vi "VI Tree.vi"   [LabVIEW 2012, in "Phidget Stepper.lvlib"]
doc: "${Stepper:VITreeHeader}"
uses:
  <instrlib>/Phidgets/Phidget Stepper/Phidget Stepper.lvlib
  <instrlib>/Phidgets/Phidget Stepper/Public/StepperStart.vi
  <instrlib>/Phidgets/Phidget Stepper/Public/StepperOpen.vi
  <instrlib>/Phidgets/Phidget Stepper/Public/StepperClose.vi
panel:
  # "(c) 2015 Phidgets Inc..  ALL RIGHTS RESERVED."
  # "SEE DIAGRAM\nFOR VI TREE."
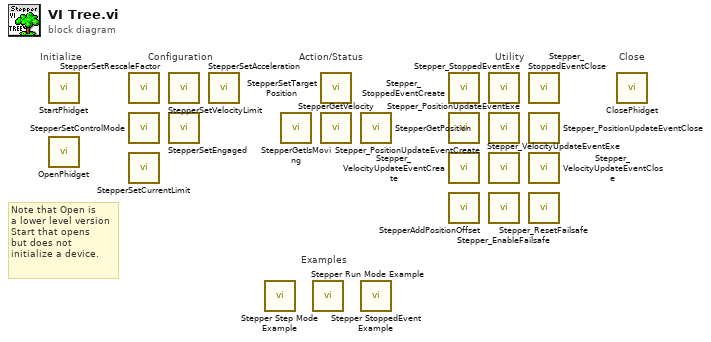
[diagram p0: block diagram]
diagram:
  # "Note that Open is\na lower level version\nStart that opens\nbut does not \ninitialize a device."
  # "Examples"
  # "Configuration"
  # "Utility"
  # "Action/Status"
  # "Close"
  # "Initialize"
  n1 = call-poly <instrlib>:"StartPhidget.vi"() -> ()  [unwired: 12 in, 4 out]
  n2 = call-poly <instrlib>:"OpenPhidget.vi"() -> ()  [unwired: 8 in, 4 out]
  n3 = call <instrlib>:"StepperSetRescaleFactor.vi"() -> ()  [unwired: 9 in, 2 out]
  n4 = call <instrlib>:"StepperSetControlMode.vi"() -> ()  [unwired: 9 in, 2 out]
  n5 = call <instrlib>:"StepperSetCurrentLimit.vi"() -> ()  [unwired: 9 in, 2 out]
  n6 = call <instrlib>:"StepperSetVelocityLimit.vi"() -> ()  [unwired: 9 in, 2 out]
  n7 = call <instrlib>:"StepperSetEngaged.vi"() -> ()  [unwired: 9 in, 2 out]
  n8 = call <instrlib>:"StepperSetAcceleration.vi"() -> ()  [unwired: 9 in, 2 out]
  n9 = call <instrlib>:"Stepper Step Mode Example.vi"() -> ()  [unwired: 12 in]
  n10 = call <instrlib>:"StepperGetIsMoving.vi"() -> ()  [unwired: 8 in, 3 out]
  n11 = call <instrlib>:"Stepper Run Mode Example.vi"() -> ()  [unwired: 12 in]
  n12 = call <instrlib>:"StepperSetTargetPosition.vi"() -> ()  [unwired: 9 in, 2 out]
  n13 = call <instrlib>:"StepperGetVelocity.vi"() -> ()  [unwired: 8 in, 3 out]
  n14 = call <instrlib>:"StepperGetPosition.vi"() -> ()  [unwired: 8 in, 3 out]
  n15 = call <instrlib>:"Stepper StoppedEvent Example.vi"() -> ()  [unwired: 12 in]
  n16 = call <instrlib>:"Stepper_StoppedEventCreate.vi"() -> ()  [unwired: 9 in, 3 out]
  n17 = call <instrlib>:"Stepper_PositionUpdateEventCreate.vi"() -> ()  [unwired: 9 in, 3 out]
  n18 = call <instrlib>:"Stepper_VelocityUpdateEventCreate.vi"() -> ()  [unwired: 9 in, 3 out]
  n19 = call <instrlib>:"StepperAddPositionOffset.vi"() -> ()  [unwired: 9 in, 2 out]
  n20 = call <instrlib>:"Stepper_StoppedEventExe.vi"() -> ()  [unwired: 6 in, 6 out]
  n21 = call <instrlib>:"Stepper_PositionUpdateEventExe.vi"() -> ()  [unwired: 5 in, 7 out]
  n22 = call <instrlib>:"Stepper_VelocityUpdateEventExe.vi"() -> ()  [unwired: 5 in, 7 out]
  n23 = call <instrlib>:"Stepper_EnableFailsafe.vi"() -> ()  [unwired: 9 in, 2 out]
  n24 = call <instrlib>:"Stepper_StoppedEventClose.vi"() -> ()  [unwired: 10 in, 2 out]
  n25 = call <instrlib>:"Stepper_PositionUpdateEventClose.vi"() -> ()  [unwired: 10 in, 2 out]
  n26 = call <instrlib>:"Stepper_VelocityUpdateEventClose.vi"() -> ()  [unwired: 10 in, 2 out]
  n27 = call <instrlib>:"Stepper_ResetFailsafe.vi"() -> ()  [unwired: 9 in, 2 out]
  n28 = call-poly <instrlib>:"ClosePhidget.vi"() -> ()  [unwired: 11 in, 1 out]
